vi "Read Trace Buffer Statistics.vi"(0 "VISA resource name":refnum<visa-resource-name>, 11 "error in (no error)":errorcluster) -> (3 "Maximum":dbl, 4 "VISA resource name out":refnum<visa-resource-name>, 6 "Peak-to-Peak":dbl, 8 "Mean":dbl, 10 "Standard Deviation":dbl, 14 "Minimum":dbl, 15 "error out":errorcluster)   [LabVIEW 2019, in "Keithley 6517.lvlib"]
doc: "Reads all the statistics of the trace buffer.\n\n<B>Note:</B>\nThis VI is comptible with both 6517 and 6514 models."
uses:
  Keithley 6517.lvlib
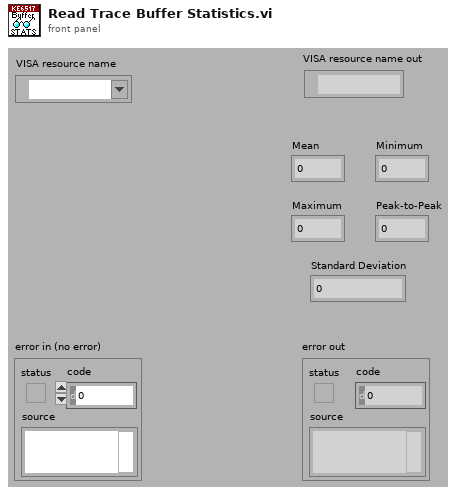
[diagram p1: front panel]
types:
  T1 = typedef "Keithley 6517.lvlib/Extended User Data.ctl" = cluster{"Instrument Model":i32}
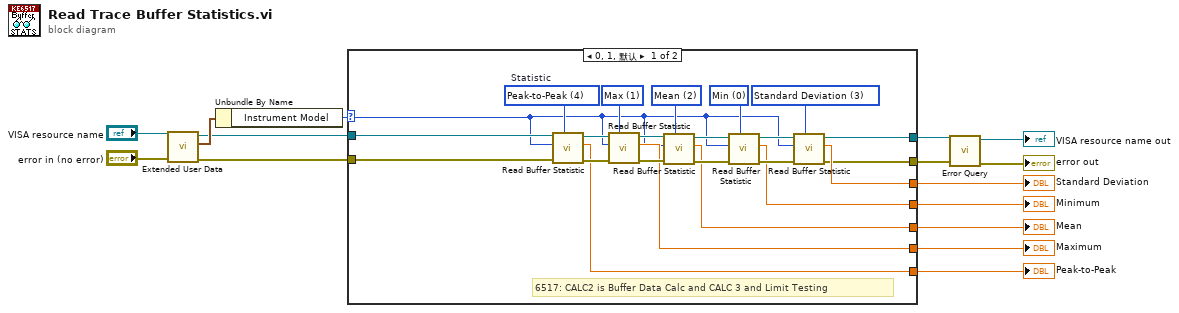
[diagram p0: block diagram]
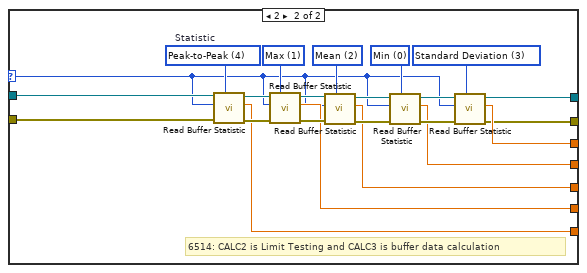
[diagram p2: hidden frame]
diagram:
  n1 = call "Extended User Data.vi"("error in (no error)"="error in (no error)", "VISA resource name"="VISA resource name") -> ("error out"=w14:errorcluster, "User Data Out"=w15:T1, "VISA resource name out"=w13:refnum<visa-resource-name>)  [unwired: 7 in]
  n2 = Unbundle By Name(w15) -> ("Instrument Model"=w10:i32)
  n3 = case shown="0, 1, 默认" w10 {
    selector: w10 -> [w16 w39]
    tunnel: w14 -> [w30 w53]
    tunnel: w13 -> [w29 w52]
    tunnel: [w23 w46] -> w9
    tunnel: [w22 w45] -> w8
    tunnel: [w21 w44] -> w7
    tunnel: [w20 w43] -> w6
    tunnel: [w19 w42] -> w5
    tunnel: [w17 w41] -> w4
    tunnel: [w18 w40] -> w3
    frame 0, 1, Default {
      w24 = 3 items=["Min", "Max", "Mean", "Standard Deviation", "Peak-to-Peak"] ("Statistic")
      w25 = 0 items=["Min", "Max", "Mean", "Standard Deviation", "Peak-to-Peak"] ("Statistic")
      w26 = 2 items=["Min", "Max", "Mean", "Standard Deviation", "Peak-to-Peak"] ("Statistic")
      w27 = 1 items=["Min", "Max", "Mean", "Standard Deviation", "Peak-to-Peak"] ("Statistic")
      w28 = 4 items=["Min", "Max", "Mean", "Standard Deviation", "Peak-to-Peak"]  # Statistic
      # "6517: CALC2 is Buffer Data Calc and CALC 3 and Limit Testing"
      n4 = call "Read Buffer Statistic.vi"("Statistic (0:Min)"=w28, "error in (no error)"=w30, "Instrument Model"=w16, "VISA resource name"=w29) -> ("error out"=w38:errorcluster, "Statistic Value"=w23:dbl, "VISA resource name out"=w37:refnum<visa-resource-name>)  [unwired: 5 in]
      n5 = call "Read Buffer Statistic.vi"("Statistic (0:Min)"=w27, "error in (no error)"=w38, "Instrument Model"=w16, "VISA resource name"=w37) -> ("error out"=w36:errorcluster, "Statistic Value"=w22:dbl, "VISA resource name out"=w35:refnum<visa-resource-name>)  [unwired: 5 in]
      n6 = call "Read Buffer Statistic.vi"("Statistic (0:Min)"=w26, "error in (no error)"=w36, "Instrument Model"=w16, "VISA resource name"=w35) -> ("error out"=w34:errorcluster, "Statistic Value"=w21:dbl, "VISA resource name out"=w33:refnum<visa-resource-name>)  [unwired: 5 in]
      n7 = call "Read Buffer Statistic.vi"("Statistic (0:Min)"=w25, "error in (no error)"=w34, "Instrument Model"=w16, "VISA resource name"=w33) -> ("error out"=w32:errorcluster, "Statistic Value"=w20:dbl, "VISA resource name out"=w31:refnum<visa-resource-name>)  [unwired: 5 in]
      n8 = call "Read Buffer Statistic.vi"("Statistic (0:Min)"=w24, "error in (no error)"=w32, "Instrument Model"=w16, "VISA resource name"=w31) -> ("error out"=w17:errorcluster, "Statistic Value"=w19:dbl, "VISA resource name out"=w18:refnum<visa-resource-name>)  [unwired: 5 in]
    }
    frame 2 {
      w47 = 3 items=["Min", "Max", "Mean", "Standard Deviation", "Peak-to-Peak"] ("Statistic")
      w48 = 0 items=["Min", "Max", "Mean", "Standard Deviation", "Peak-to-Peak"] ("Statistic")
      w49 = 2 items=["Min", "Max", "Mean", "Standard Deviation", "Peak-to-Peak"] ("Statistic")
      w50 = 1 items=["Min", "Max", "Mean", "Standard Deviation", "Peak-to-Peak"] ("Statistic")
      w51 = 4 items=["Min", "Max", "Mean", "Standard Deviation", "Peak-to-Peak"]  # Statistic
      # "6514: CALC2 is Limit Testing and CALC3 is buffer data calculation"
      n9 = call "Read Buffer Statistic.vi"("Statistic (0:Min)"=w51, "error in (no error)"=w53, "Instrument Model"=w39, "VISA resource name"=w52) -> ("error out"=w61:errorcluster, "Statistic Value"=w46:dbl, "VISA resource name out"=w60:refnum<visa-resource-name>)  [unwired: 5 in]
      n10 = call "Read Buffer Statistic.vi"("Statistic (0:Min)"=w50, "error in (no error)"=w61, "Instrument Model"=w39, "VISA resource name"=w60) -> ("error out"=w59:errorcluster, "Statistic Value"=w45:dbl, "VISA resource name out"=w58:refnum<visa-resource-name>)  [unwired: 5 in]
      n11 = call "Read Buffer Statistic.vi"("Statistic (0:Min)"=w49, "error in (no error)"=w59, "Instrument Model"=w39, "VISA resource name"=w58) -> ("error out"=w57:errorcluster, "Statistic Value"=w44:dbl, "VISA resource name out"=w56:refnum<visa-resource-name>)  [unwired: 5 in]
      n12 = call "Read Buffer Statistic.vi"("Statistic (0:Min)"=w48, "error in (no error)"=w57, "Instrument Model"=w39, "VISA resource name"=w56) -> ("error out"=w55:errorcluster, "Statistic Value"=w43:dbl, "VISA resource name out"=w54:refnum<visa-resource-name>)  [unwired: 5 in]
      n13 = call "Read Buffer Statistic.vi"("Statistic (0:Min)"=w47, "error in (no error)"=w55, "Instrument Model"=w39, "VISA resource name"=w54) -> ("error out"=w41:errorcluster, "Statistic Value"=w42:dbl, "VISA resource name out"=w40:refnum<visa-resource-name>)  [unwired: 5 in]
    }
  }
  "Peak-to-Peak" <- w9
  "Maximum" <- w8
  "Mean" <- w7
  "Minimum" <- w6
  "Standard Deviation" <- w5
  n14 = call "Error Query.vi"("error in (no error)"=w4, "VISA resource name"=w3) -> ("error out"=→"error out":errorcluster, "VISA resource name out"=→"VISA resource name out":refnum<visa-resource-name>)  [unwired: 6 in, 2 out]
